vi "libssh2_sftp_readlink.vi"(7 "maxlen":u32, 8 "error in (no error)":errorcluster, 10 "path":string, 11 "sftp":T1) -> (0 "error out":errorcluster, 2 "target":string)   [LabVIEW 2017, in "libssh2.lvlib"]
doc: "Read the target of a symbolic link."
uses:
  libssh2.lvlib
  SFTP Refnum.ctl
  libssh2_sftp_symlink_type.ctl
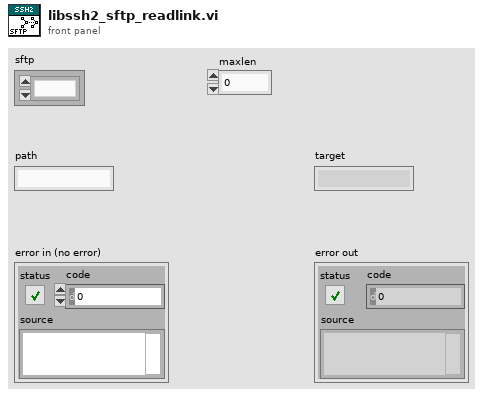
[diagram p1: front panel]
types:
  T1 = typedef "libssh2.lvlib/SFTP Refnum.ctl" = refnum<k1>
  T2 = typedef "libssh2.lvlib/libssh2_sftp_symlink_type.ctl" = enum16{"SYMLINK", "READLINK", "REALPATH"}
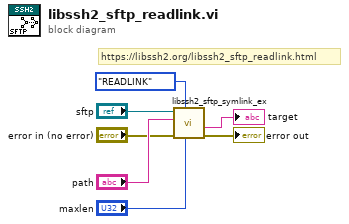
[diagram p0: block diagram]
diagram:
  # "https://libssh2.org/libssh2_sftp_readlink.html"
  n1 = call "libssh2_sftp_symlink_ex.vi"("target_len"="maxlen", "link_type"=libssh2_sftp_symlink_type."READLINK" ("link type"), "error in (no error)"="error in (no error)", "path"="path", "sftp"="sftp") -> ("error out"=→"error out":errorcluster, "target out"=→"target":string)  [unwired: 5 in]
